vi "Actor Core.vi"(8 "error in":errorcluster, 11 "Data Saver in":refnum<class "Data Saver.lvclass">) -> (0 "error out":errorcluster, 3 "Actor out":refnum<class "Actor.lvclass">)   [LabVIEW 2014, in "Data Saving.lvlib" / "Data Saver.lvclass"]
doc: "(<B>Filename</B>: Actor Framework.lvlib:Actor.lvclass:Actor Core.vi)\n\nReceives messages to the actor, reacts to them, and initiates any error handling that may shut the actor down.\n\nDescendant classes may override this VI to append parallel tasks for the actor to complete while it handles messages. Overrides use the Call Parent Method node."
uses:
  Data Saver.lvclass
  <vilib>/ActorFramework/Actor/Actor.lvclass
  <vilib>/express/express shared/transition.llb/Dynamic To Waveform Array.vi
  <vilib>/express/express signal manip/GetorSetDDTAttributes/Set DDT Attributes/SetT0.vi
  <vilib>/express/express shared/transition.llb/Waveform Array To Dynamic.vi
  <vilib>/express/express signal manip/GetorSetDDTAttributes/Set DDT Attributes/Set DDT Properties.xnode
panel:
  in  "Waveform Graph":dynamicdata(graph)
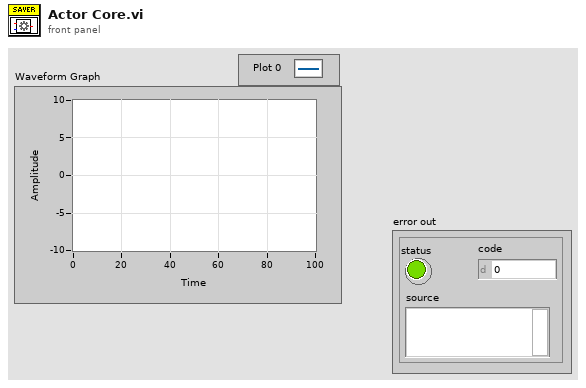
[diagram p1: front panel]
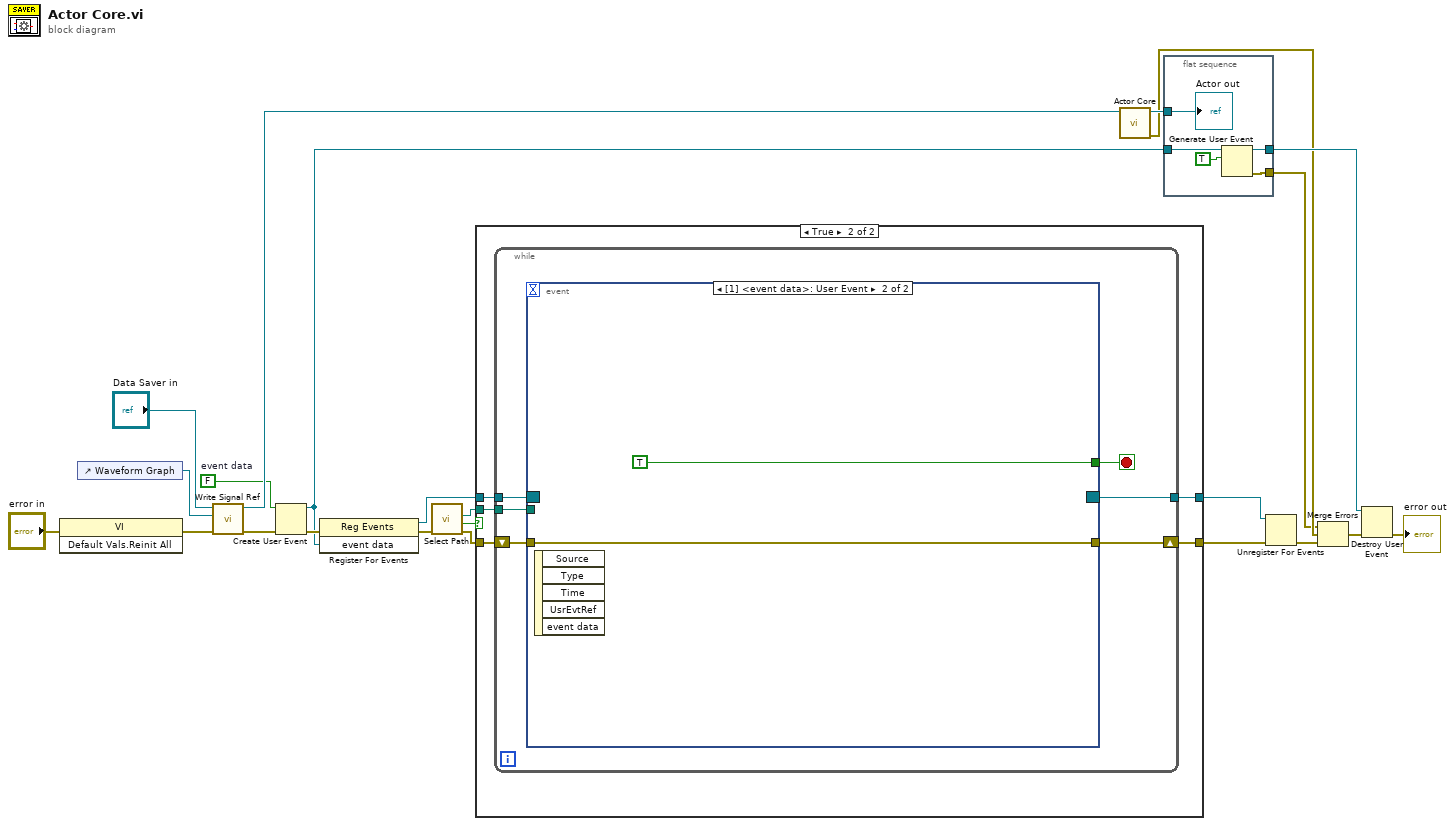
[diagram p0: block diagram]
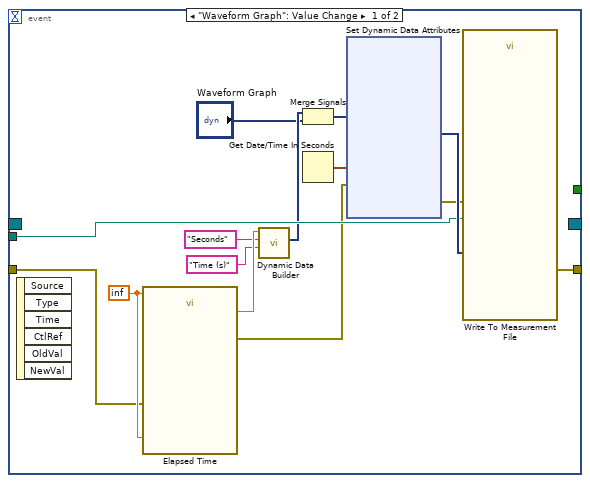
[diagram p3: hidden frame]
diagram:
  w16 = FALSE  # event data
  n1 = invoke class="VI" method="Default Vals.Reinit All"(error in="error in") -> (error out=w19:errorcluster)  [unwired: 2 in, 2 out]
  n2 = control-ref of="Waveform Graph"() -> (w18:refnum<vi>)
  n3 = call-dynamic "Write Signal Ref.vi"("error in (no error)"=w19, "Signal Ref"=w18, "Data Saver in"="Data Saver in") -> ("error out"=w15:errorcluster, "Data Saver out"=w21:refnum<class "Data Saver.lvclass">)  [unwired: 7 in]
  n4 = Create User Event(user event datatype=w16, error in=w15) -> (user event=w12:refnum<user-event>, error out=w17:errorcluster)
  n5 = register-events(error in=w17, w12) -> (reference out=w11:refnum<event-registration>, error out=w14:errorcluster)  [unwired: 1 in]
  n6 = call "Select Path.vi"("error in"=w14) -> ("error out"=w4:errorcluster, "Save?"=w13:bool, "selected path"=w2:path)  [unwired: 7 in, 1 out]
  n7 = case shown="True" w13 {
    tunnel: w11 -> [w25 w30]
    tunnel: [w25 w29] -> w8
    tunnel: w4 -> [w24 w28]
    tunnel: [w24 w27] -> w3
    tunnel: w2 -> [_ w26]
    frame False {
    }
    frame True {
      n8 = while {
        tunnel: w30 -> [w36]
        tunnel: [w35] -> w29
        shift-right: [w31] -> w27
        shift-left: w28 -> [w32]
        tunnel: w26 -> [w33]
        stop <- w34 stop-if-true
        n9 = event shown="[1] <event data>: User Event" {
          selector: w36 -> [_ _]
          dyn-events: [_ _] -> w35
          timeout: _ -> [_ _]
          tunnel: [_ TRUE] -> w34
          tunnel: w33 -> [w46 _]
          tunnel: w32 -> [w42 w65]
          tunnel: [w37 w65] -> w31
          event "Waveform Graph": Value Change {
            w43 = inf
            n10 = event-data() -> ()  [unwired: 1 in, 6 out]
            n11 = call "Elapsed Time"("Time Target (s)"=w43, "error in (no error)"=w42, "Set Start Time (s)"=w43) -> ("Elapsed Time (s)"=w41:dbl, "error out"=w38:errorcluster)  [unwired: 9 in, 6 out]
            n12 = call "Dynamic Data Builder.vi"("Signal Name"="Time (s)", "Unit"="Seconds", "Number in"=w41) -> ("Dynamic Signame Out"=w45:dynamicdata)  [unwired: 8 in]
            n13 = Merge Signals(w45, "Waveform Graph") -> (w50:dynamicdata)
            n14 = Get Date/Time In Seconds() -> (seconds since 1Jan1904=w48:timestamp)
            n15 = xnode "Set Dynamic Data Attributes"("Signals In"=w50, "Timestamp"=w48, "error in"=w38) -> ("Signals Out"=w49:dynamicdata, "error out"=w47:errorcluster)  [unwired: 1 in]
            n16 = call "Write To Measurement File"("Signals"=w49, "error in (no error)"=w47, "Filename"=w46) -> ("error out"=w37:errorcluster)  [unwired: 14 in, 2 out]
          }
          event User Event {
            n17 = event-data() -> ()  [unwired: 1 in, 5 out]
          }
        }
      }
    }
  }
  n18 = call-parent "Actor Core.vi"("Actor in"=w21) -> ("error out"=w6:errorcluster, "Actor out"=w23:refnum<class "Actor.lvclass">)  [unwired: 9 in]
  n19 = flat-sequence {
    tunnel: w23 -> [w71]
    tunnel: w12 -> [w70]
    tunnel: [w68] -> w5
    tunnel: [w67] -> w7
    frame #0 {
      n20 = Generate User Event(user event=w70, event data cluster=TRUE ("event data")) -> (user event out=w67:refnum<user-event>, error out=w68:errorcluster)  [unwired: 2 in]
      "Actor out" <- w71
    }
  }
  n21 = Unregister For Events(event registration refnum=w8, error in=w3) -> (error out=w10:errorcluster)
  n22 = Merge Errors(w5, w6, w10) -> (w9:errorcluster)
  n23 = Destroy User Event(user event=w7, error in=w9) -> (error out=→"error out":errorcluster)
